vi "from string.vi"(8 "error in":errorcluster, 9 "data":string, 10 "version":string, 11 "configuration in":refnum<class "PL_System Configuration.lvclass">) -> (0 "error out":errorcluster, 3 "configuration out":refnum<class "PL_System Configuration.lvclass">)   [LabVIEW 2013, in "PL_System Configuration.lvclass"]
doc: "Provides an interface for loading a module configuration from a file or other serialized data source. It is recommended that all children of this class store data in two sets--data required for its own initialization, and any data required for parent initialization--and that each implementation uses the <b>Call Parent Method</b> primitive to de-serialize parent information."
uses:
  PL_System Configuration.lvclass
  PL_System Configuration.lvclass/PL_System Configuration.ctl
  <vilib>/NI/Tag Bus Module Framework/root configuration/TBM configuration.lvclass
  <vilib>/NI/Configuration Framework/serializable configuration/NISE_CEF_serializable configuration.lvclass
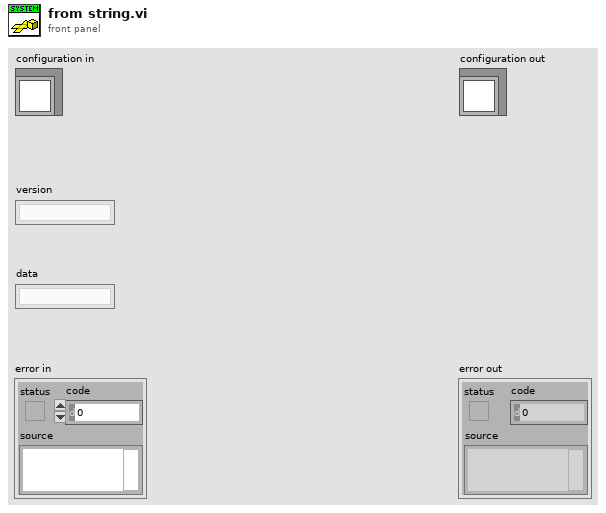
[diagram p1: front panel]
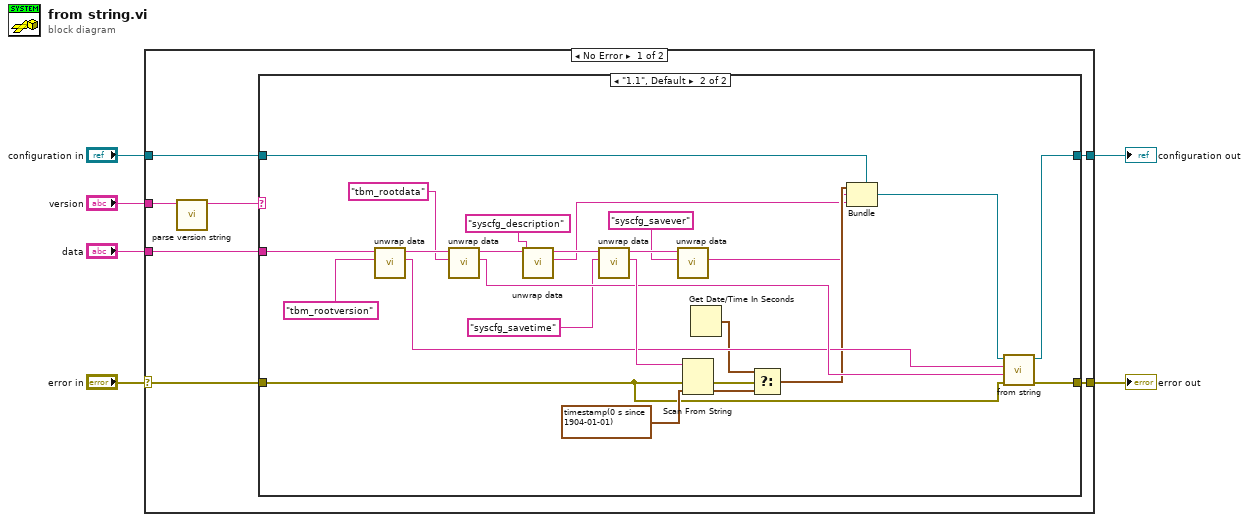
[diagram p0: block diagram]
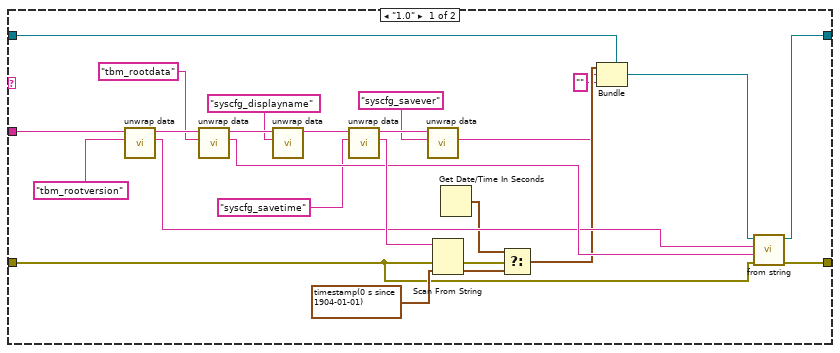
[diagram p2: hidden frame]
diagram:
  n1 = case shown="No Error" "error in" {
    selector: "error in" -> [w8 w65]
    tunnel: "data" -> [w13 _]
    tunnel: "configuration in" -> [w12 w64]
    tunnel: [w11 w64] -> w1
    tunnel: [w7 w65] -> w2
    tunnel: "version" -> [w10 _]
    frame No Error {
      n2 = call <vilib>:"parse version string.vi"("full version"=w10) -> ("major.minor version"=w9:string)  [unwired: 7 in, 3 out]
      n3 = case shown="\"1.1\", Default" w9 {
        tunnel: w13 -> [w37 w62]
        tunnel: w8 -> [w20 w45]
        tunnel: w12 -> [w38 w63]
        tunnel: [w34 w59] -> w11
        tunnel: [w36 w61] -> w7
        frame "1.0" {
          n4 = call <vilib>:"unwrap data.vi"("identifier"="tbm_rootversion" ("additional identifier"), "data to unwrap"=w37) -> ("unwrapped data"=w27:string, "remaining string"=w30:string)  [unwired: 8 in]
          n5 = call <vilib>:"unwrap data.vi"("identifier"="tbm_rootdata" ("additional identifier"), "data to unwrap"=w30) -> ("unwrapped data"=w28:string, "remaining string"=w31:string)  [unwired: 8 in]
          n6 = call <vilib>:"unwrap data.vi"("identifier"="syscfg_displayname" ("additional identifier"), "data to unwrap"=w31) -> ("remaining string"=w32:string)  [unwired: 8 in, 1 out]
          n7 = call <vilib>:"unwrap data.vi"("identifier"="syscfg_savetime" ("additional identifier"), "data to unwrap"=w32) -> ("unwrapped data"=w29:string, "remaining string"=w22:string)  [unwired: 8 in]
          n8 = call <vilib>:"unwrap data.vi"("identifier"="syscfg_savever" ("additional identifier"), "data to unwrap"=w22) -> ("unwrapped data"=w15:string)  [unwired: 8 in, 1 out]
          n9 = Scan From String(input string=w29, error in=w20, default 1=timestamp(0 s since 1904-01-01)) -> (error out=w18:errorcluster, output 1=w19:timestamp)  [unwired: 2 in, 2 out]
          n10 = Get Date/Time In Seconds() -> (seconds since 1Jan1904=w17:timestamp)
          n11 = Select(t=w17, s=w18, f=w19) -> (s? t:f=w16:timestamp)
          n12 = Bundle(cluster=w38, w16, w15, "" ("description")) -> (w35:refnum<class "PL_System Configuration.lvclass">)
          n13 = call-parent "from string.vi"("error in"=w20, "data"=w28, "version"=w27, "configuration in"=w35) -> ("error out"=w36:errorcluster, "configuration out"=w34:refnum<class "PL_System Configuration.lvclass">)  [unwired: 6 in]
        }
        frame "1.1", Default {
          n14 = call <vilib>:"unwrap data.vi"("identifier"="tbm_rootversion" ("additional identifier"), "data to unwrap"=w62) -> ("unwrapped data"=w52:string, "remaining string"=w55:string)  [unwired: 8 in]
          n15 = call <vilib>:"unwrap data.vi"("identifier"="tbm_rootdata" ("additional identifier"), "data to unwrap"=w55) -> ("unwrapped data"=w53:string, "remaining string"=w56:string)  [unwired: 8 in]
          n16 = call <vilib>:"unwrap data.vi"("identifier"="syscfg_description" ("additional identifier"), "data to unwrap"=w56) -> ("unwrapped data"=w39:string, "remaining string"=w57:string)  [unwired: 8 in]
          n17 = call <vilib>:"unwrap data.vi"("identifier"="syscfg_savetime" ("additional identifier"), "data to unwrap"=w57) -> ("unwrapped data"=w54:string, "remaining string"=w47:string)  [unwired: 8 in]
          n18 = call <vilib>:"unwrap data.vi"("identifier"="syscfg_savever" ("additional identifier"), "data to unwrap"=w47) -> ("unwrapped data"=w40:string)  [unwired: 8 in, 1 out]
          n19 = Scan From String(input string=w54, error in=w45, default 1=timestamp(0 s since 1904-01-01)) -> (error out=w43:errorcluster, output 1=w44:timestamp)  [unwired: 2 in, 2 out]
          n20 = Get Date/Time In Seconds() -> (seconds since 1Jan1904=w42:timestamp)
          n21 = Select(t=w42, s=w43, f=w44) -> (s? t:f=w41:timestamp)
          n22 = Bundle(cluster=w63, w41, w40, w39) -> (w60:refnum<class "PL_System Configuration.lvclass">)
          n23 = call-parent "from string.vi"("error in"=w45, "data"=w53, "version"=w52, "configuration in"=w60) -> ("error out"=w61:errorcluster, "configuration out"=w59:refnum<class "PL_System Configuration.lvclass">)  [unwired: 6 in]
        }
      }
    }
    frame Error {
    }
  }
  "error out" <- w2
  "configuration out" <- w1
